vi "ftngen.vi"() -> ()   [LabVIEW 2019]
panel:
  in  "Amplitude":dbl(knob) scale=0.0..10.0
  in  "frequency":dbl(knob) scale=0.0..10.0
  out "Waveform Graph":waveform(dbl)(graph)
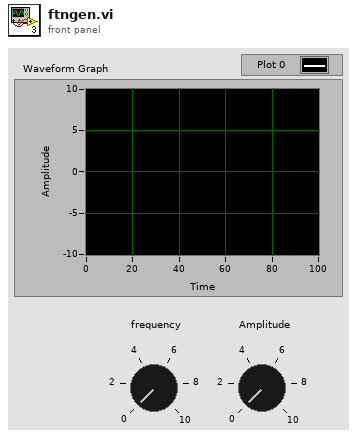
[diagram p1: front panel]
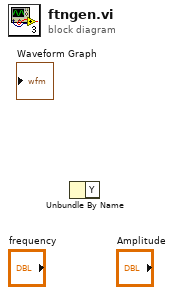
[diagram p0: block diagram]
diagram:
  n1 = Unbundle By Name() -> ()  [unwired: 1 in, 1 out]
